vi "Update-map-data.vi"(4 "Active characteristic":T1, 6 "Active camera":T2, 8 "error in":errorcluster, 10 "Storage params. ref.":refnum<data-value>, 11 "Mapping params. ref. in":refnum<data-value>) -> (0 "error IO":errorcluster, 2 "Map":T3, 3 "Mapping params. ref.":refnum<data-value>)   [LabVIEW 2013, in "CameraVision.lvlib" / "CV-Mapping.lvclass"]
uses:
  CV-Mapping.lvclass
  Storage/CV-Storage.lvclass
  UI/Camera-selector.ctl
  Mapping-characteristic.ctl
  Storage/CV-Storage.lvclass/CV-Storage.ctl
  CV-Mapping.lvclass/CV-Mapping.ctl
  Read Time.vi
  Read Xcoors.vi
  Read Ycoors.vi
  Read Scan start.vi
  Storage/Read Characteristics file reference RO.vi
  Storage/Read Temperature file reference W.vi
  Storage/Read Camera suffix.vi
  UI/CV-UI.lvclass
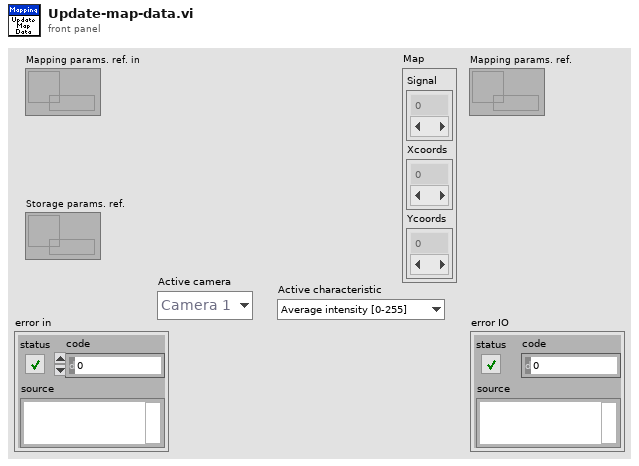
[diagram p1: front panel]
types:
  T1 = typedef "CameraVision.lvlib/CV-Mapping.lvclass/Mapping-characteristic.ctl" = enum16{"Average intensity [0-255]", "Peak intensity [0-255]", "Melt-pool size [mm²]", "Melt-pool aspect ratio []", "Melt-pool fragments []", "Average temperature [°C]", "Max. temperature [°C]", "Min. temperature [°C]", "Std. dev. temperature [°C]"}
  T2 = typedef "CameraVision.lvlib/CV-UI.lvclass/Camera-selector.ctl" = enum16{"Camera 1", "Camera 2"}
  T3 = cluster{"Signal":sgl[], "Xcoords":sgl[], "Ycoords":sgl[]}
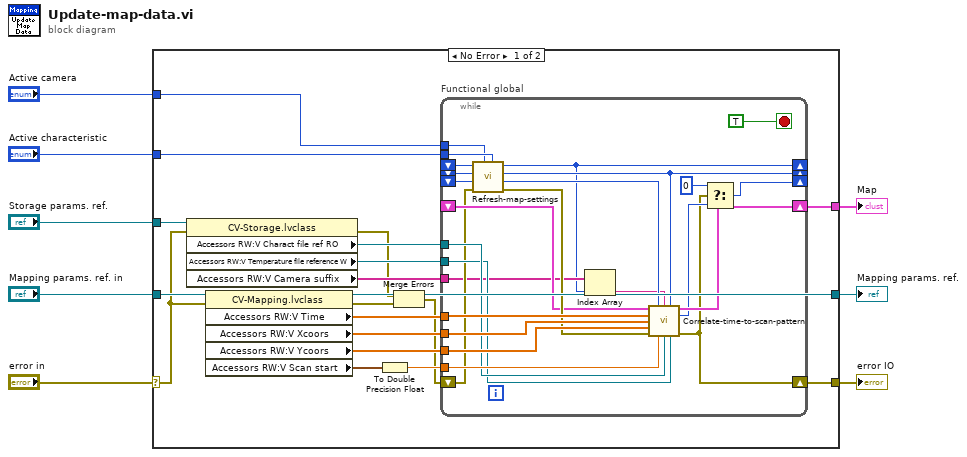
[diagram p0: block diagram]
diagram:
  n1 = case shown="No Error" "error in" {
    selector: "error in" -> [w11 w54]
    tunnel: [w27 w54] -> w8
    tunnel: "Mapping params. ref. in" -> [w25 w53]
    tunnel: [w20 w53] -> w5
    tunnel: "Storage params. ref." -> [w19 _]
    tunnel: [w15 _] -> w3
    tunnel: "Active characteristic" -> [w10 _]
    tunnel: "Active camera" -> [w9 _]
    frame No Error {
      n2 = property class="CV-Storage.lvclass"(reference=w19, error in=w11) -> (error out=w12:errorcluster, "Accessors RW:V Charact file ref RO"=w18:refnum<k34>, "Accessors RW:V Temperature file reference W"=w17:refnum<k34>, "Accessors RW:V Camera suffix"=w16:string[])  [unwired: 1 out]
      n3 = property class="CV-Mapping.lvclass"(reference=w25, error in=w11) -> (reference out=w20:refnum<data-value>, error out=w14:errorcluster, "Accessors RW:V Time"=w24:sgl[], "Accessors RW:V Xcoors"=w23:sgl[], "Accessors RW:V Ycoors"=w22:sgl[], "Accessors RW:V Scan start"=w21:timestamp)
      n4 = To Double Precision Float(number=w21) -> (double precision float=w26:dbl)
      n5 = Merge Errors(w12, w14) -> (w13:errorcluster)
      n6 = while "Functional global" {
        shift-right: [w32] -> w27
        shift-left: w13 -> [w37]
        shift-right: [w43] -> _
        shift-left: _ -> [w51]
        shift-right: [w33] -> _
        shift-left: _ -> [w50]
        shift-right: [w28] -> _
        shift-left: _ -> [w52]
        tunnel: w26 -> [w44]
        tunnel: w24 -> [w48]
        tunnel: w23 -> [w47]
        tunnel: w22 -> [w46]
        tunnel: w18 -> [w39]
        tunnel: w17 -> [w38]
        tunnel: w16 -> [w29]
        shift-right: [w40] -> w15
        shift-left: _ -> [w41]
        tunnel: w10 -> [w31]
        tunnel: w9 -> [w30]
        stop <- TRUE stop-if-true
        n7 = call "Refresh-map-settings.vi"("Active characteristic"=w31, "Active camera"=w30, "error in"=w37, "Read offset buffer in"=w50, "Map characteristic buffer in"=w51, "Active camer buffer in"=w52) -> ("error IO"=w45:errorcluster, "Read offset"=w49:i64, "Map characteristic"=w43:T1, "Active camera"=w28:T2)  [unwired: 1 in, 1 out]
        n8 = Index Array(array=w29, index=w28) -> (element=w42:string)
        n9 = call "Correlate-time-to-scan-pattern.vi"("Map in"=w41, "Read offset"=w49, "Camera"=w42, "Map characteristic"=w43, "Pattern time"=w48, "Pattern X"=w47, "Pattern Y"=w46, "error in"=w45, "Scan start time [s]"=w44, "Characteristics file ref."=w39, "Temperature file ref."=w38) -> ("Map"=w40:T3, "New offset"=w35:i64, "error IO"=w32:errorcluster)  [unwired: 2 in]
        n10 = Select(t=i64 0, s=w32, f=w35) -> (s? t:f=w33:i64)
      }
    }
    frame Error {
    }
  }
  "error IO" <- w8
  "Mapping params. ref." <- w5
  "Map" <- w3
